vi "Get ini file value.vi"(0 "configuration file path":path, 5 "section":string, 7 "key":string, 9 "String/Number":bool, 11 "error in (no error)":errorcluster) -> (4 "String value":string, 6 "Numeric value":u32, 15 "error out":errorcluster)   [LabVIEW 2025]
uses:
  <vilib>/Utility/config.llb/Read Key (U32).vi
  <vilib>/Utility/config.llb/Read Key (String).vi
  <vilib>/Utility/config.llb/NI_LVConfig.lvlib
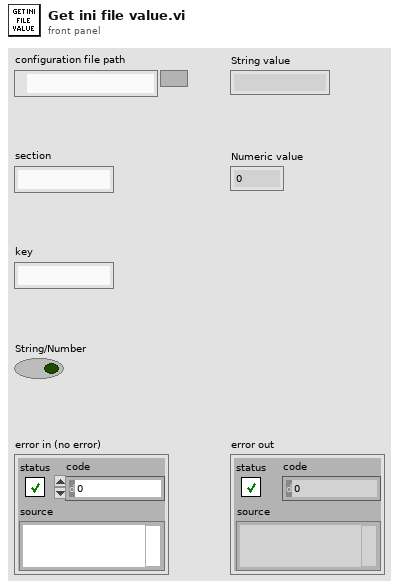
[diagram p1: front panel]
types:
  T1 = typedef "NI_LVConfig.lvlib/Config Data RefNum.ctl" = refnum<k1>
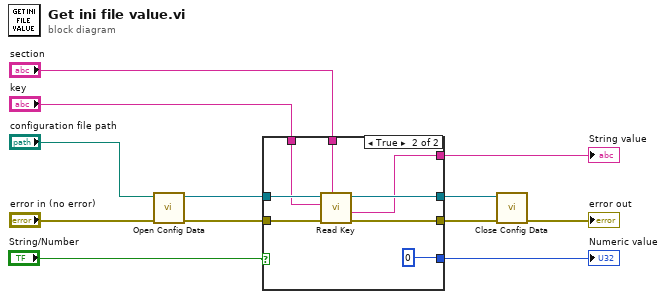
[diagram p0: block diagram]
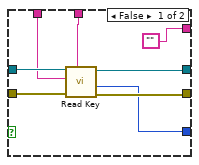
[diagram p2: hidden frame]
diagram:
  n1 = call <vilib>:"Open Config Data.vi"("error in (no error)"="error in (no error)", "configuration file path"="configuration file path") -> ("error out"=w9:errorcluster, "refnum"=w10:T1)  [unwired: 7 in, 1 out]
  n2 = case shown="True" "String/Number" {
    tunnel: w10 -> [w20 w28]
    tunnel: w9 -> [w19 w27]
    tunnel: [w18 w26] -> w8
    tunnel: [w17 w25] -> w7
    tunnel: "section" -> [w14 w24]
    tunnel: "key" -> [w15 w23]
    tunnel: ["" w22] -> w4
    tunnel: [w16 u32 0 ("value")] -> w2
    frame False {
      n3 = call-poly <vilib>:"Read Key.vi"("section"=w14, "error in (no error)"=w19, "key"=w15, "refnum"=w20) -> ("error out"=w17:errorcluster, "value"=w16:u32, "refnum out"=w18:T1)  [unwired: 4 in, 1 out]
    }
    frame True {
      n4 = call-poly <vilib>:"Read Key.vi"("section"=w24, "error in (no error)"=w27, "key"=w23, "refnum"=w28) -> ("error out"=w25:errorcluster, "value"=w22:string, "refnum out"=w26:T1)  [unwired: 4 in, 1 out]
    }
  }
  "String value" <- w4
  "Numeric value" <- w2
  n5 = call <vilib>:"Close Config Data.vi"("error in (no error)"=w7, "refnum"=w8) -> ("error out"=→"error out":errorcluster)  [unwired: 8 in, 1 out]
